vi "getViBlockDiagram.vi"(6 "closeVIRef":bool, 8 "error in (no error)":errorcluster, 11 "ViRef":refnum<vi>) -> (0 "error out":errorcluster, 3 "topMostBlockDiagram":refnum<class "BlockDiagram.lvclass">)   [LabVIEW 2023, in "TLC_Scripto.lvlib"]
uses:
  TLC_Scripto.lvlib
  BlockDiagram/BlockDiagram.lvclass
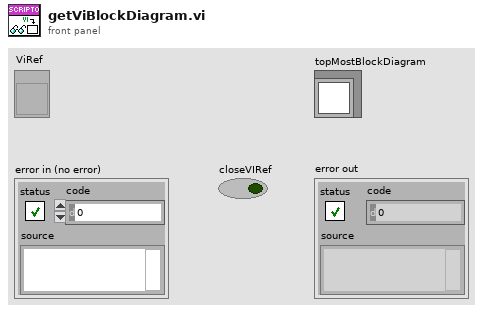
[diagram p1: front panel]
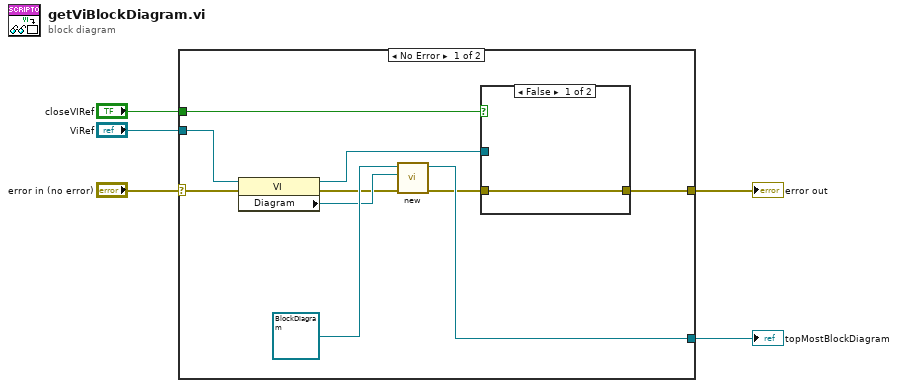
[diagram p0: block diagram]
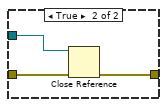
[diagram p2: hidden frame]
diagram:
  n1 = case shown="No Error" "error in (no error)" {
    selector: "error in (no error)" -> [w6 w20]
    tunnel: "ViRef" -> [w8 _]
    tunnel: [w12 _] -> w2
    tunnel: [w10 w20] -> w3
    tunnel: "closeVIRef" -> [w7 _]
    frame No Error {
      n2 = property class="VI"(reference=w8, error in=w6) -> (reference out=w9:refnum<vi>, error out=w13:errorcluster, "Diagram"=w14:refnum<vi>)
      n3 = call-dynamic "new.vi"("Error In"=w13, "ref"=w14, "GObject in"=refnum<class "BlockDiagram.lvclass"> refnum ("TLC_Scripto.lvlib:BlockDiagram.lvclass")) -> ("Error Out"=w11:errorcluster, "GObject out"=w12:refnum<class "BlockDiagram.lvclass">)  [unwired: 7 in]
      n4 = case shown="False" w7 {
        tunnel: w11 -> [w16 w19]
        tunnel: [w16 w18] -> w10
        tunnel: w9 -> [_ w17]
        frame False {
        }
        frame True {
          n5 = Close Reference(reference=w17, error in (no error)=w19) -> (error out=w18:errorcluster)
        }
      }
    }
    frame Error {
    }
  }
  "error out" <- w3
  "topMostBlockDiagram" <- w2
